vi "Test Array Send.vi"(7 "LabVIEW Web Service Request":refnum<class "Web Request.lvclass">, 10 "num":dbl, 11 "DataIn":dbl[](array[numeric])) -> ()   [LabVIEW 2014]
uses:
  <vilib>/wsapi/Web Request.lvclass
panel:
  out "Array - Numeric 2":dbl[](array[numeric])
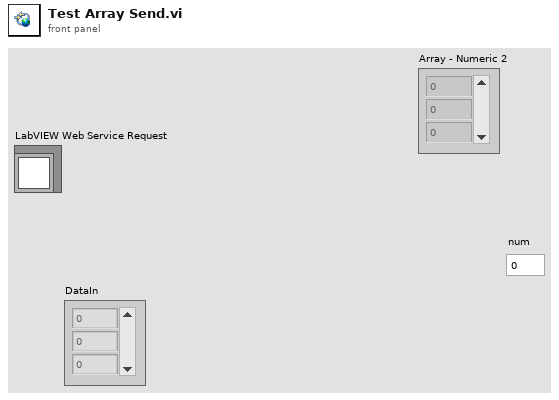
[diagram p1: front panel]
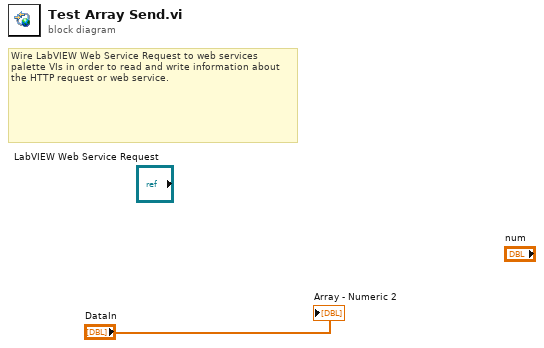
[diagram p0: block diagram]
diagram:
  # "Wire LabVIEW Web Service Request to web services palette VIs in order to read and write information about the HTTP request or web service."
  "Array - Numeric 2" <- "DataIn"
